vi "Registered UIMsg Codes.vi"() -> (3 "UIMessage Codes":T1[](array[typedef])=[enum."Trace"])   [LabVIEW 2020, in "TSnax.lvlib" / "Execution.lvclass"]
uses:
  Execution.lvclass
  Execution.lvclass/Execution.ctl
  UIMsg.ctl
  TSnax.lvlib
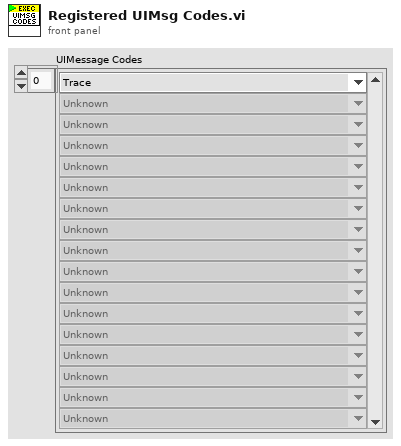
[diagram p1: front panel]
types:
  T1 = typedef "TSnax.lvlib/UIMsg.ctl" = enum16{"Unknown", "BreakOnUserRequest", "BreakOnBreakpoint", "BreakOnRunTimeError", "Trace", "TerminatingExecution", "AbortingExecution", "KillingExecutionThreads", "EndExecution", "ShutDownComplete", "StartExecution", "ProgressPercent", "ProgressText", "StartInteractiveExecution", "EndInteractiveExecution", "TerminatingInteractiveExecution", "TerminationCancelled", "ResumeFromBreak", "StartFileExecution", "EndFileExecution", "ShutDownCancelled", "LocalizationSettingChanged", "OpenWindows", "TileWindows", "CascadeWindows", "ReportChanged", "CloseWindows", "RefreshWindows", "ClientFileChanged", "DisplayReport", "ModelState_Initializing", "ModelState_Waiting", "ModelState_Identified", "ModelState_BeginTesting", "ModelState_TestingComplete", "ModelState_PostProcessingComplete", "ModelState_EnabledStateSet", "ReportLocationChanged", "GotoLocation", "PushUndoItem", "OutputMessages", "TypePaletteFileListChanged", "NonTerminatingThreadsArePreventingTermination", "ModelState_PostProcessing", "ReportCollectionChanged", "RuntimeError"}
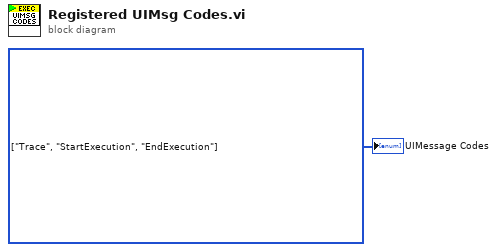
[diagram p0: block diagram]
diagram:
  w1 = T1[] [enum."Trace", enum."StartExecution", enum."EndExecution"] items=["Unknown", "BreakOnUserRequest", "BreakOnBreakpoint", "BreakOnRunTimeError", "Trace", "TerminatingExecution", "AbortingExecution", "KillingExecutionThreads", "EndExecution", "ShutDownComplete", "StartExecution", "ProgressPercent", "ProgressText", "StartInteractiveExecution", "EndInteractiveExecution", "TerminatingInteractiveExecution", "TerminationCancelled", "ResumeFromBreak", "StartFileExecution", "EndFileExecution", "ShutDownCancelled", "LocalizationSettingChanged", "OpenWindows", "TileWindows", "CascadeWindows", "ReportChanged", "CloseWindows", "RefreshWindows", "ClientFileChanged", "DisplayReport", "ModelState_Initializing", "ModelState_Waiting", "ModelState_Identified", "ModelState_BeginTesting", "ModelState_TestingComplete", "ModelState_PostProcessingComplete", "ModelState_EnabledStateSet", "ReportLocationChanged", "GotoLocation", "PushUndoItem", "OutputMessages", "TypePaletteFileListChanged", "NonTerminatingThreadsArePreventingTermination", "ModelState_PostProcessing", "ReportCollectionChanged", "RuntimeError"] ("UIMessage IDs")
  "UIMessage Codes" <- w1
